vi "Start Command.vi"(8 "error in (no error)":errorcluster, 11 "Command in":refnum<class "Drive by Power.lvclass">) -> (0 "error out":errorcluster, 3 "Command out":refnum<class "Drive by Power.lvclass">)   [LabVIEW 2014, in "Forward Drive.lvlib" / "Drive by Power.lvclass"]
uses:
  Drive by Power.lvclass
  Drive by Power.lvclass/Drive by Power.ctl
  Forward Drive Messages/Set Power Msg/Set Power Msg.lvclass/Set Power Msg.ctl
  <vilib>/ActorFramework/Message Enqueuer/Message Enqueuer.lvclass/Message Enqueuer.ctl
  <vilib>/ActorFramework/Actor/Actor.lvclass/Actor.ctl
  <vilib>/ActorFramework/Message Enqueuer/Enqueue.vi
  <vilib>/ActorFramework/Message Enqueuer/Init from Existing Queue.vi
  <vilib>/ActorFramework/Message Priority Queue/Priority Enqueue.vi
  <vilib>/ActorFramework/Message Enqueuer/Message Enqueuer.lvclass
  Robot Actor Framework/Command Actor/Command Actor Messages/FInished Command Msg/Finish Command Msg.lvclass
  Forward Drive Messages/Set Power Msg/Set Power Msg.lvclass
  Forward Drive Cmd.lvclass
  <vilib>/ActorFramework/Actor/Actor.lvclass
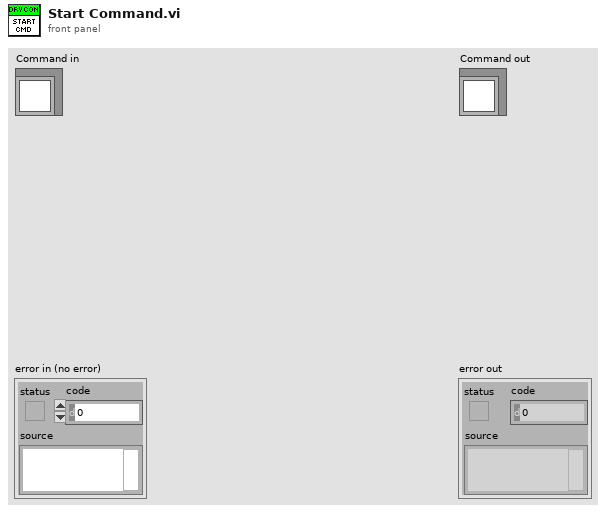
[diagram p1: front panel]
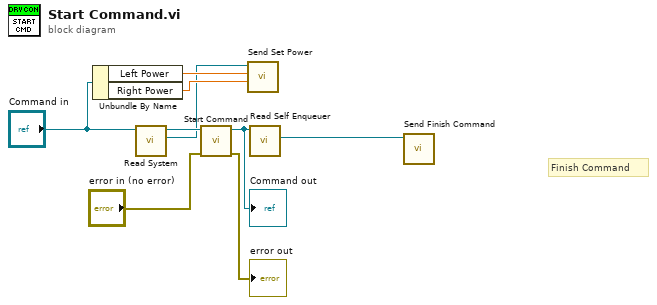
[diagram p0: block diagram]
diagram:
  # "Finish Command"
  n1 = Unbundle By Name("Command in") -> ("Left Power"=w7:dbl, "Right Power"=w6:dbl)
  n2 = call-dynamic "Read System.vi"("Command in"="Command in") -> ("Actor Framework:Message Enqueuer"=w1:refnum<class "Message Enqueuer.lvclass">, "Command out"=w2:refnum<class "Drive by Power.lvclass">)  [unwired: 8 in, 1 out]
  n3 = call-parent "Start Command.vi"("error in (no error)"="error in (no error)", "Command in"=w2) -> ("error out"=→"error out":errorcluster, "Command out"=w5:refnum<class "Drive by Power.lvclass">)  [unwired: 8 in]
  "Command out" <- w5
  n4 = call "Send Set Power.vi"("Right Power"=w6, "Left Power"=w7, "Message Enqueuer"=w1) -> ()  [unwired: 7 in, 2 out]
  n5 = call <vilib>:"Read Self Enqueuer.vi"("Actor"=w5) -> ("Self Enqueuer"=w4:refnum<class "Message Enqueuer.lvclass">)  [unwired: 10 in]
  n6 = call "Send Finish Command.vi"("Message Enqueuer"=w4) -> ()  [unwired: 9 in, 2 out]
